vi "grap display.vi"(8 "error in":errorcluster, 11 "file path (dialog if empty)":path) -> (0 "error out":errorcluster, 3 "XY GRAPH":cluster{"X":dbl[], "Y":dbl[]}[](array[cluster]))   [LabVIEW 2023]
uses:
  <vilib>/Utility/file.llb/Read Delimited Spreadsheet (string).vi
panel:
  out "XY Graph 2":cluster{"X":dbl[], "Y":dbl[]}[](graph)
  out "TEMP":string[](array[string])
  out "COF":string[](array[string])
  out "TIME":string[](array[string])
  out "all rows":string[][](array[string])
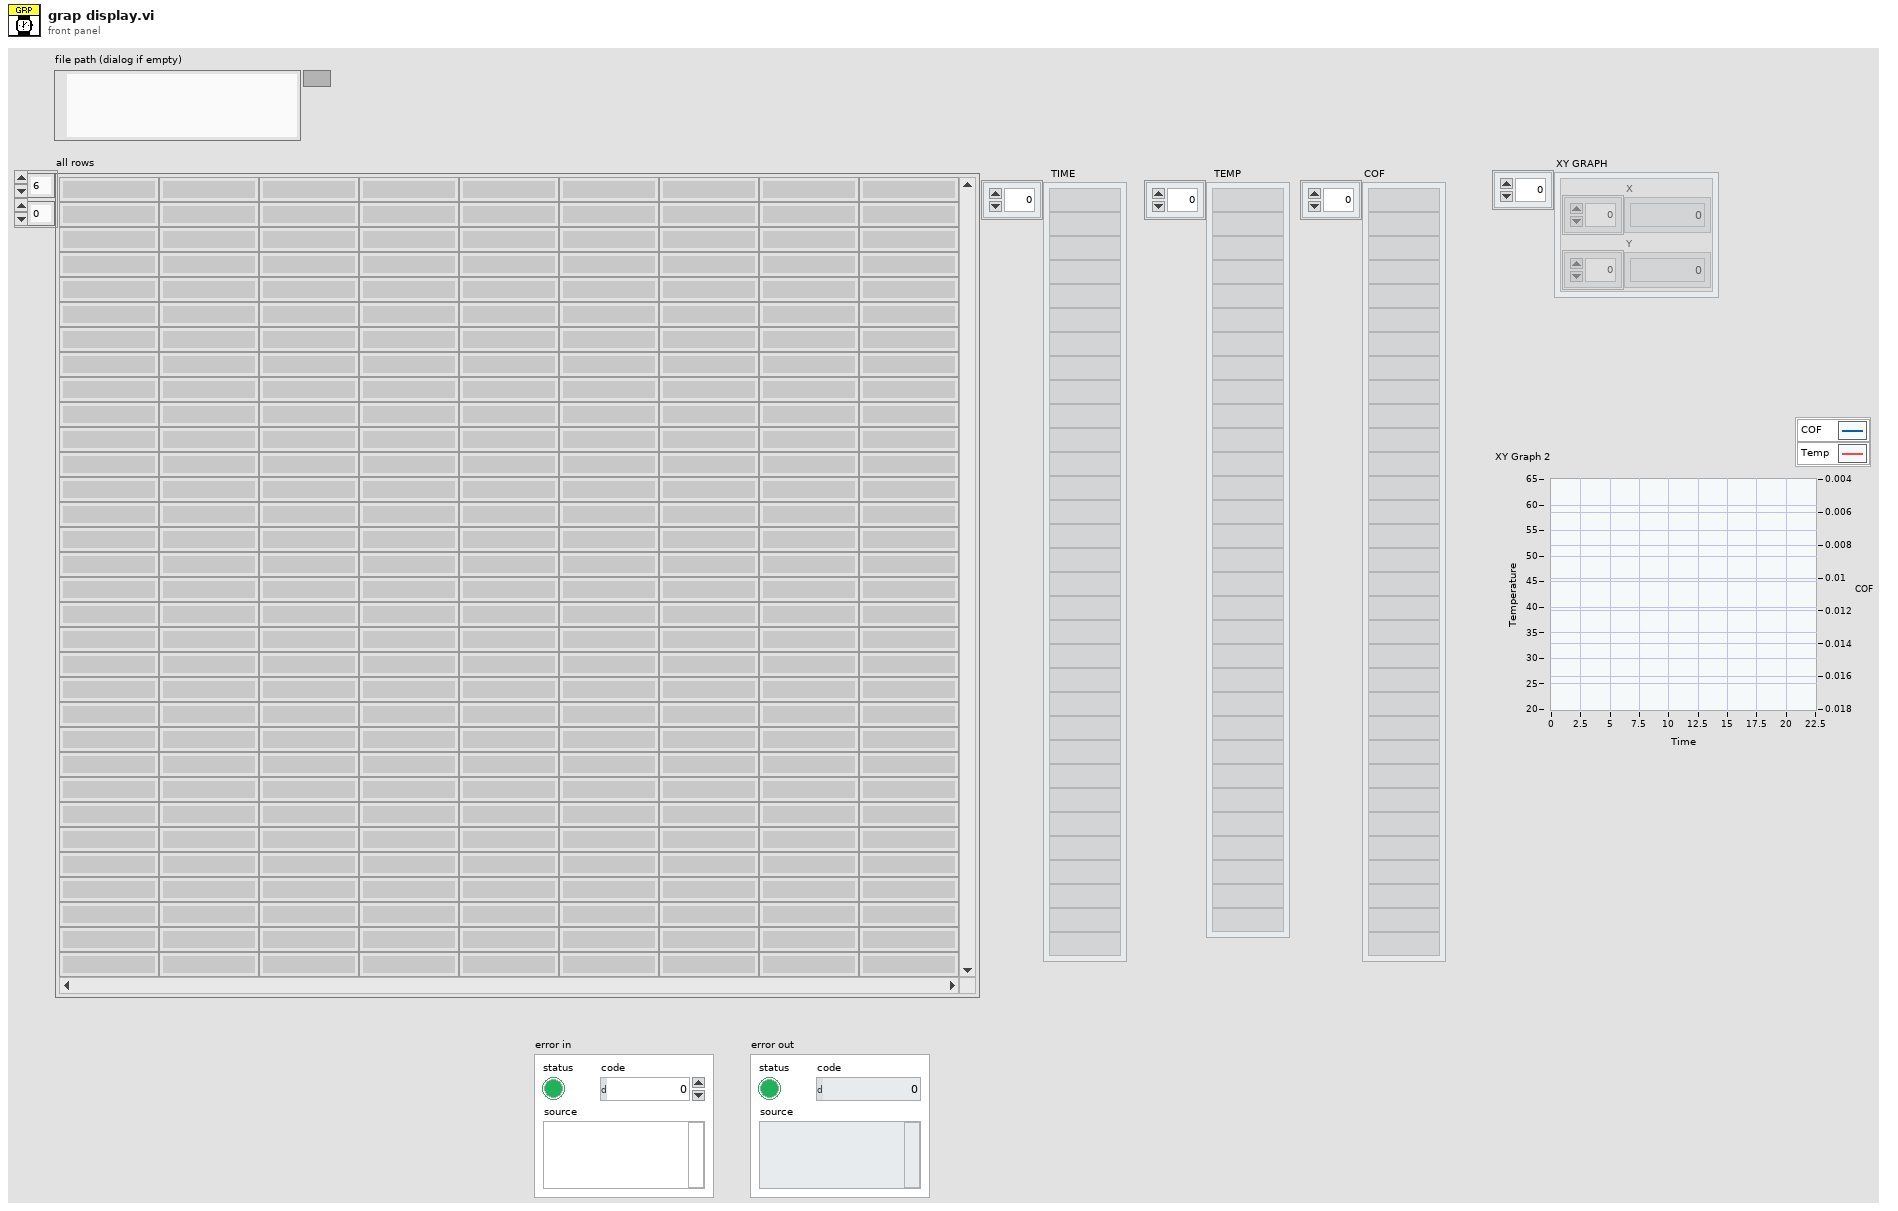
[diagram p1: front panel]
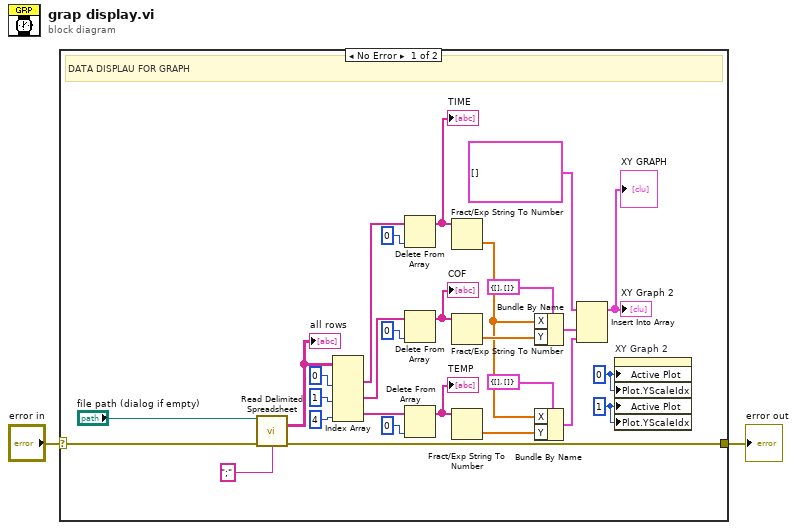
[diagram p0: block diagram]
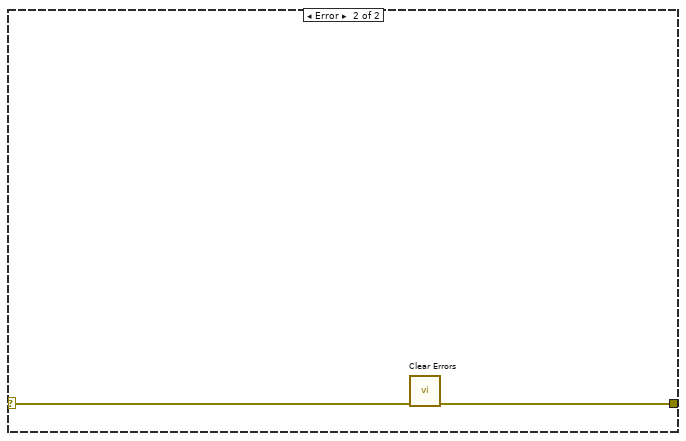
[diagram p2: hidden frame]
diagram:
  n1 = case shown="No Error" "error in" {
    selector: "error in" -> [w6 w32]
    tunnel: [w5 w31] -> w1
    frame No Error {
      w3 = u32 1 ("Active Plot")
      w4 = u32 0 ("Active Plot")
      # "DATA DISPLAU FOR GRAPH"
      n2 = call-poly <vilib>:"Read Delimited Spreadsheet.vi"("file path (dialog if empty)"="file path (dialog if empty)", "error in (no error)"=w6, "delimiter (\\t)"=";" ("delimiter (\\t)")) -> ("all rows"=w28:string[][], "error out"=w5:errorcluster)  [unwired: 7 in, 4 out]
      "all rows" <- w28
      n3 = Index Array(array=w28, index (col) #1=0 ("disabled index (col)"), index (col) #2=1 ("index (col)"), index (col) #3=4 ("index (col)")) -> (element #1=w16:string[], element #2=w10:string[], element #3=w15:string[])  [unwired: 3 in]
      n4 = Delete From Array(array=w16, index=0) -> (array with subset deleted=w11:string[])  [unwired: 1 in, 1 out]
      "TIME" <- w11
      n5 = Delete From Array(array=w10, index=0) -> (array with subset deleted=w9:string[])  [unwired: 1 in, 1 out]
      "COF" <- w9
      n6 = Delete From Array(array=w15, index=0) -> (array with subset deleted=w8:string[])  [unwired: 1 in, 1 out]
      "TEMP" <- w8
      n7 = Fract/Exp String To Number(string=w11) -> (number=w19:dbl[])  [unwired: 3 in, 1 out]
      n8 = Fract/Exp String To Number(string=w9) -> (number=w21:dbl[])  [unwired: 3 in, 1 out]
      n9 = Fract/Exp String To Number(string=w8) -> (number=w18:dbl[])  [unwired: 3 in, 1 out]
      n10 = Bundle By Name(cluster=cluster{"X":dbl[], "Y":dbl[]} {"X"=[], "Y"=[]} ("new element/subarray"), "X"=w19, "Y"=w21) -> (w23:cluster{"X":dbl[], "Y":dbl[]})
      n11 = Bundle By Name(cluster=cluster{"X":dbl[], "Y":dbl[]} {"X"=[], "Y"=[]} ("new element/subarray"), "X"=w19, "Y"=w18) -> (w17:cluster{"X":dbl[], "Y":dbl[]})
      n12 = Insert Into Array(array=cluster{"X":dbl[], "Y":dbl[]}[] [] ("XY Graph"), new element #1=w23, new element #2=w17) -> (→"XY Graph 2" →"XY GRAPH":cluster{"X":dbl[], "Y":dbl[]}[])  [unwired: 1 in]
      n13 = property on="XY Graph 2" class="XYGraph (strict)"("Active Plot"=w4, "Plot.YScaleIdx"=w4, "Active Plot"=w3, "Plot.YScaleIdx"=w3) -> ()  [unwired: 2 in, 2 out]
    }
    frame Error {
      n14 = call <vilib>:"Clear Errors.vi"("error in (no error)"=w32) -> ("error out"=w31:errorcluster)  [unwired: 5 in, 1 out]
    }
  }
  "error out" <- w1
